vi "Node_ID_AlarmAck.vi"(8 "error in":errorcluster) -> (0 "error out":errorcluster, 1 "node RU 3":string[](array[string]), 2 "node RU 2":T1[](array[typedef]), 3 "node RU":T1[](array[typedef]))   [LabVIEW 2019]
uses:
  <vilib>/OPCUA/controls/NodeId.ctl
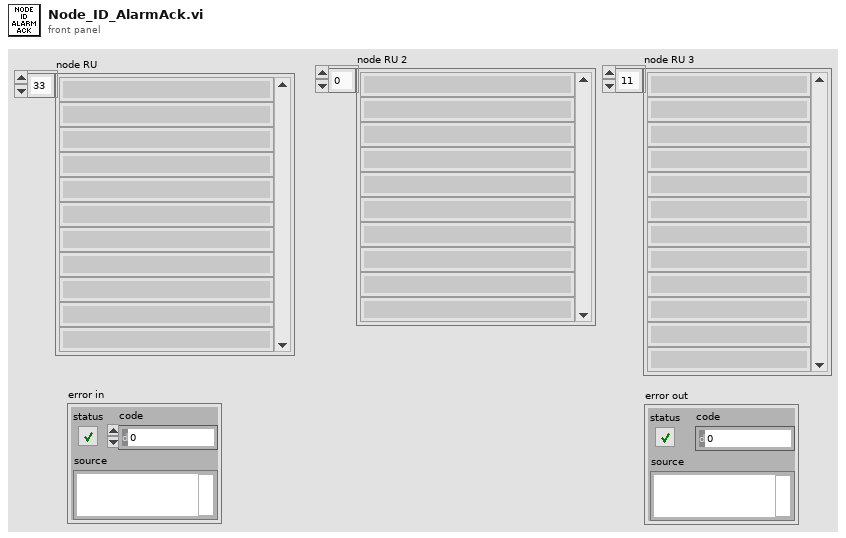
[diagram p1: front panel]
types:
  T1 = typedef "NodeId.ctl" = string
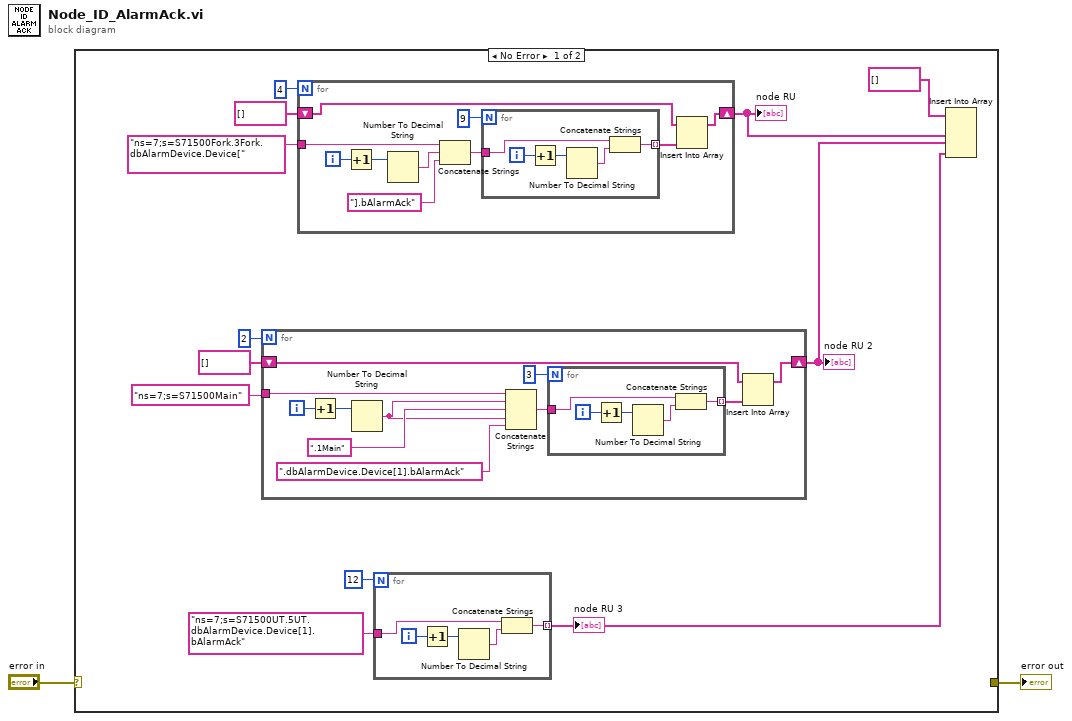
[diagram p0: block diagram]
diagram:
  n1 = case shown="No Error" "error in" {
    selector: "error in" -> [_ w51]
    tunnel: [_ w51] -> w1
    frame No Error {
      n2 = for {
        N: 2 -> [_]
        tunnel: T1 "ns=7;s=S71500Main" ("node RU") -> [w29]
        shift-right: [w26] -> w4
        shift-left: T1[] [] ("node RU") -> [w24]
        i -> [w28]
        n3 = Increment(x=w28) -> (x+1=w30:i32)
        n4 = Number To Decimal String(number=w30) -> (decimal integer string=w22:string)  [unwired: 1 in]
        n5 = Concatenate Strings(w29, w22, ".1Main" ("string"), w22, ".dbAlarmDevice.Device[1].bAlarmAck" ("string")) -> (w27:string)
        n6 = for {
          N: 3 -> [_]
          tunnel: w27 -> [w35]
          tunnel: [w31] -> w25 mode=indexing
          i -> [w34]
          n7 = Increment(x=w34) -> (x+1=w33:i32)
          n8 = Number To Decimal String(number=w33) -> (decimal integer string=w32:string)  [unwired: 1 in]
          n9 = Concatenate Strings(w35, w32) -> (w31:string)
        }
        n10 = Insert Into Array(array=w24, new element=w25) -> (w26:T1[])  [unwired: 1 in]
      }
      "node RU 2" <- w4
      n11 = for {
        N: 4 -> [_]
        tunnel: T1 "ns=7;s=S71500Fork.3Fork.dbAlarmDevice.Device[" ("node RU") -> [w43]
        shift-right: [w38] -> w5
        shift-left: T1[] [] ("node RU") -> [w36]
        i -> [w42]
        n12 = Increment(x=w42) -> (x+1=w45:i32)
        n13 = Number To Decimal String(number=w45) -> (decimal integer string=w44:string)  [unwired: 1 in]
        n14 = Concatenate Strings(w43, w44, "].bAlarmAck" ("string")) -> (w39:string)
        n15 = for {
          N: 9 -> [_]
          tunnel: w39 -> [w50]
          tunnel: [w46] -> w37 mode=indexing
          i -> [w49]
          n16 = Increment(x=w49) -> (x+1=w48:i32)
          n17 = Number To Decimal String(number=w48) -> (decimal integer string=w47:string)  [unwired: 1 in]
          n18 = Concatenate Strings(w50, w47) -> (w46:string)
        }
        n19 = Insert Into Array(array=w36, new element=w37) -> (w38:T1[])  [unwired: 1 in]
      }
      "node RU" <- w5
      n20 = for {
        N: 12 -> [_]
        tunnel: T1 "ns=7;s=S71500UT.5UT.dbAlarmDevice.Device[1].bAlarmAck" ("node RU") -> [w19]
        tunnel: [w15] -> w3 mode=indexing
        i -> [w18]
        n21 = Increment(x=w18) -> (x+1=w17:i32)
        n22 = Number To Decimal String(number=w17) -> (decimal integer string=w16:string)  [unwired: 1 in]
        n23 = Concatenate Strings(w19, w16) -> (w15:string)
      }
      "node RU 3" <- w3
      n24 = Insert Into Array(array=T1[] [] ("node RU"), new element #1=w5, new element #2=w4, new element #3=w3) -> ()  [unwired: 1 in, 1 out]
    }
    frame Error {
    }
  }
  "error out" <- w1
